vi "未命名 2.vi"() -> ()   [LabVIEW 2013]
uses:
  C:/Program Files (x86)/National Instruments/LabVIEW 2013/examples/Controls and Indicators/XControls/Dual Mode Thermometer/Simple Dual Mode Thermometer XControl.xctl
panel:
  in  "停止":bool
  in  "简单双模式温度计XControl":dbl(xcontrol)
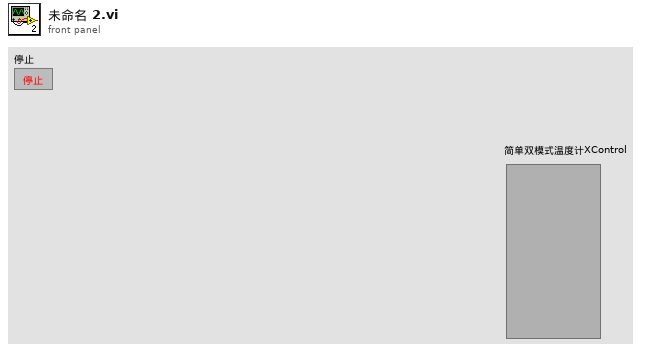
[diagram p1: front panel]
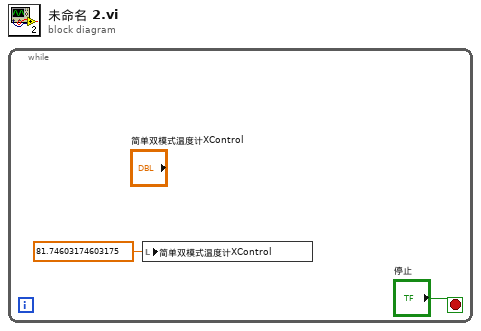
[diagram p0: block diagram]
diagram:
  n1 = while {
    stop <- "停止" stop-if-true
    n2 = local write "简单双模式温度计XControl"(81.74603174603175 ("简单双模式温度计XControl")) -> ()
  }
